vi "server.vi"() -> ()   [LabVIEW 2013, in "Experiment.lvclass"]
uses:
  Experiment.lvclass
  HSDIO/HSDIO_settings.ctl
  <instrlib>/niHSDIO/niHSDIO.llb/niHSDIO_ctl Trigger Script - trigID Values (Ring).ctl
  <instrlib>/niHSDIO/niHSDIO.llb/niHSDIO_ctl Trigger Source Values (Ring).ctl
  <instrlib>/niHSDIO/niHSDIO.llb/niHSDIO_ctl Trigger DigEdge - Edge Values (Ring).ctl
  <instrlib>/niHSDIO/niHSDIO.llb/niHSDIO_ctl Trigger DigLvl - Level Values (Ring).ctl
  HSDIO/waveform.ctl
  Camera/Hamamatsu_C9100-13/camera_setup.ctl
  <vilib>/Platform/TimedLoop/XDataNode/timing_clust.ctl
  <vilib>/Platform/TimedLoop/XDataNode/nitl_modes.ctl
  <vilib>/Platform/TimedLoop/XDataNode/wakeup.ctl
  Experiment.lvclass/Experiment.ctl
  HSDIO/HSDIO.lvclass
  Camera/Hamamatsu_C9100-13/Hamamatsu_C9100-13.lvclass
  Globals.vi
  <vilib>/platform/TimedLoop/XDataNode/XDataNode.xnode
  TCP_IP/TCP_IP.lvclass
  <vilib>/Platform/TimedLoop/XDataNode/XDNodeRunTimeDep.lvlib
panel:
  out "Log History":string
  in  "Tab Control":enum32{"HSDIO", "Camera"}(tab)=enum."Camera"
  out "HSDIO Settings":T1={"Enable HSDIO Pulses"=FALSE, "Resource Name"="PXI1Slot6", "Clock Rate"=20000000.0, "Array of Script Triggers"=[], "Pulse Generation Script"="script script1\n     Generate RedTrap_compress_temp\nend script", "Start Trigger"={"Wait for start trigger?"=FALSE, "source (PFI 0)"="PFI0", "edge (rising)"=12}, "Hardware alignment quantum\n(in samples)"=1, "Inital State"="", "Idle State"="", "Active Channels"="", "Array of Waveforms"=[]} {"Hardware alignment quantum\n(in samples)" min=1 step=1; "Array of Script Triggers"."level" items=["High Level"=34, "Low Level"=35]; "Array of Script Triggers"."edge" items=["Rising Edge"=12, "Falling Edge"=13]; "Start Trigger"."edge (rising)" items=["Rising Edge"=12, "Falling Edge"=13]; "Clock Rate" min=0.0 max=200000000.0 format="%.2p"}
  out "Camera Setup":T7={"Analog Gain (0-5)"=0, "Exposure Time"=0.01, "EM Gain (0-255)"=0, "Trigger Polarity"="ATP P", "External Trigger Mode"="EMD E", "Scan Speed"="SSP H", "External Trigger Source"="ESC B", "Scan Mode"="SMD N", "Super Pixel Binning\n(if enabled in Scan Mode)"="SPX 1", "Camera Sub-array acquisition region\n(if enabled in scan mode)"={"Left"=0, "Top"=0, "Width"=0, "Height"=0}, "Use camera?"=FALSE, "# image buffers"=100, "shots per measurement"=2, "Force images to U16"=FALSE, "Low Light Sensitivity"="LLS 0", "cooling"="CSW F", "fan"="FAN F", "Frame Grabber acquisition region"={"Left"=0, "Top"=0, "Right"=0, "Bottom"=0}} {"Frame Grabber acquisition region"."Bottom" max=512 step=1; "Frame Grabber acquisition region"."Right" max=512 step=1; "Frame Grabber acquisition region"."Top" max=512 step=1; "Frame Grabber acquisition region"."Left" max=512 step=1; "shots per measurement" min=0 step=1; "# image buffers" min=0 step=1; "Camera Sub-array acquisition region\n(if enabled in scan mode)"."Height" min=16 max=512 step=16; "Camera Sub-array acquisition region\n(if enabled in scan mode)"."Width" min=16 max=512 step=16; "Camera Sub-array acquisition region\n(if enabled in scan mode)"."Top" max=496 step=16; "Camera Sub-array acquisition region\n(if enabled in scan mode)"."Left" max=496 step=16; "Analog Gain (0-5)" max=5 step=1}
  in  "Clear Log":bool
  in  "Return fake test data":bool=TRUE
  out "Done":bool
  in  "Restart":bool
  out "Log":string
  in  "Stop":bool
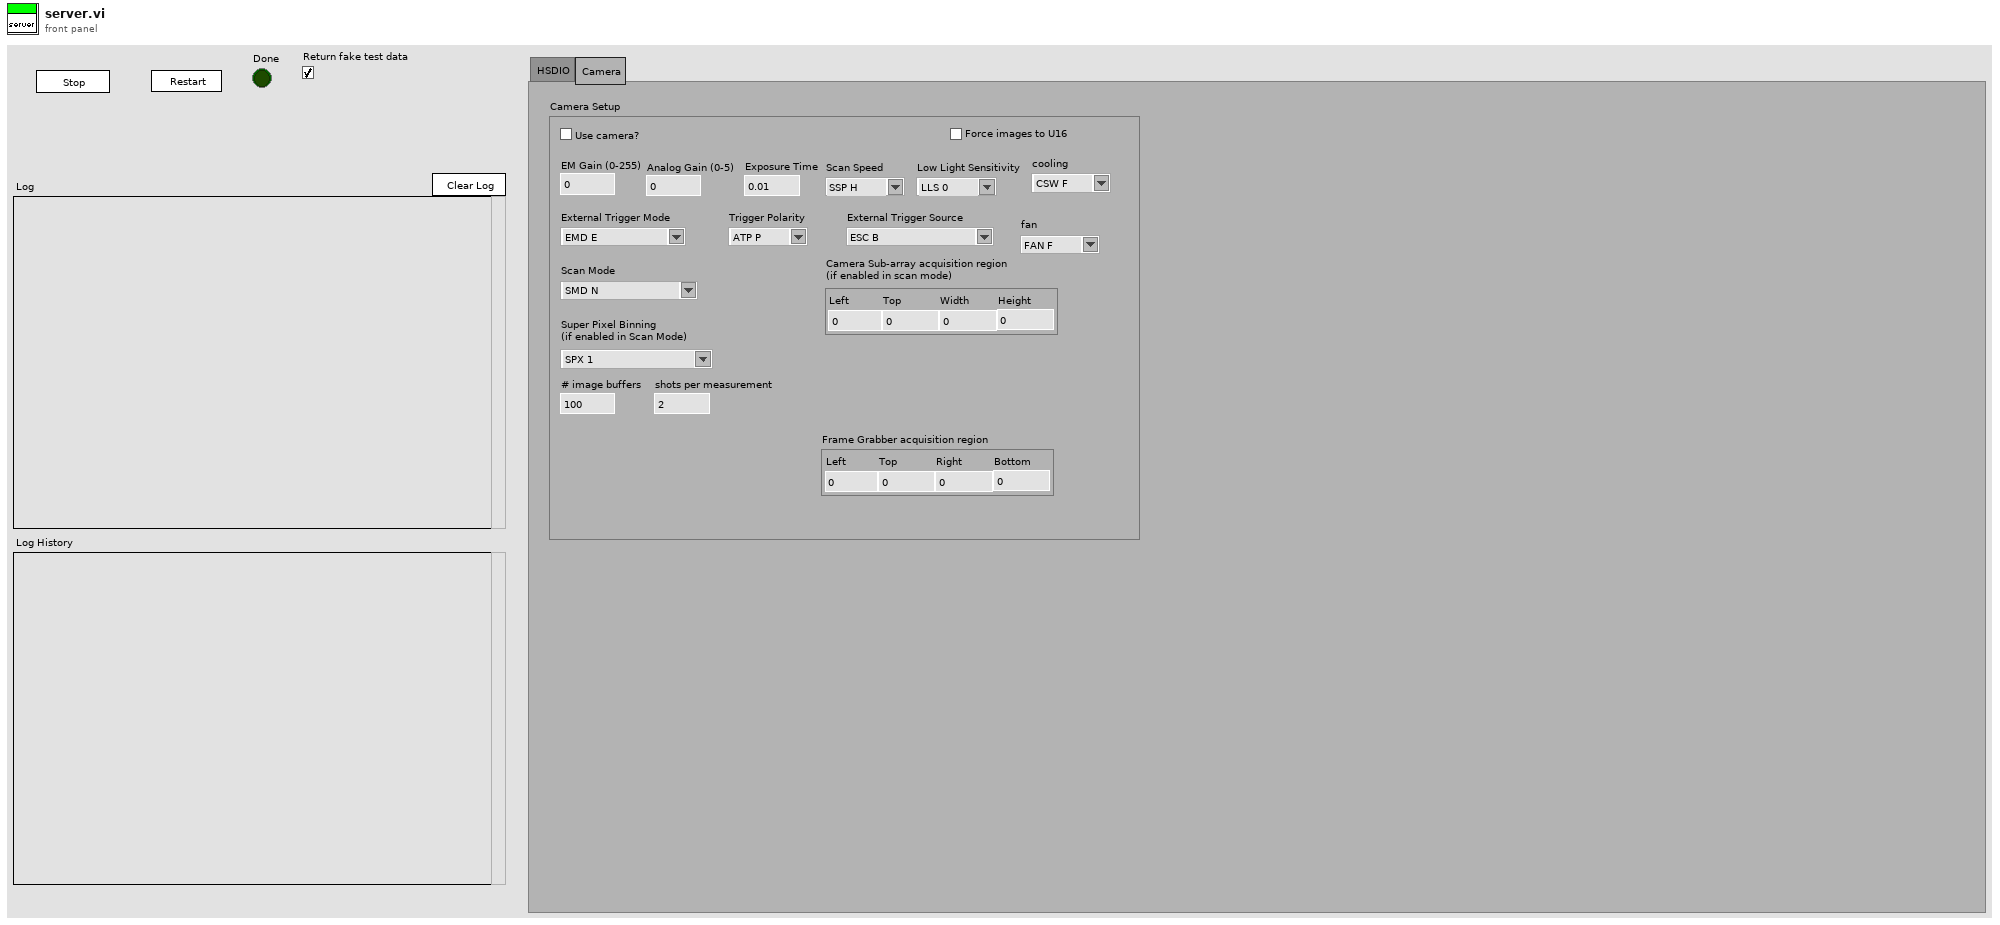
[diagram p1: front panel]
types:
  T1 = typedef "HSDIO.lvclass/HSDIO_settings.ctl" = cluster{"Enable HSDIO Pulses":bool, "Resource Name":refnum<k15>, "Clock Rate":dbl, "Array of Script Triggers":cluster{"trigger id (script trigger 0)":T2, "source (PFI 0)":T3, "Trigger Type":enum32{"Edge", "Level"}, "edge":T4, "level":T5}[], "Pulse Generation Script":string, "Start Trigger":cluster{"Wait for start trigger?":bool, "source (PFI 0)":T3, "edge (rising)":T4}, "Hardware alignment quantum\n(in samples)":u16, "Inital State":string, "Idle State":string, "Active Channels":string, "Array of Waveforms":T6[]}
  T2 = typedef "niHSDIO_ctl Trigger Script - trigID Values (Ring).ctl" = string
  T3 = typedef "niHSDIO_ctl Trigger Source Values (Ring).ctl" = string
  T4 = typedef "niHSDIO_ctl Trigger DigEdge - Edge Values (Ring).ctl" = i32
  T5 = typedef "niHSDIO_ctl Trigger DigLvl - Level Values (Ring).ctl" = i32
  T6 = typedef "HSDIO.lvclass/waveform.ctl" = cluster{"name":string, "transitions":u32[], "states":u8[][]}
  T7 = typedef "Hamamatsu_C9100-13.lvclass/camera_setup.ctl" = cluster{"Analog Gain (0-5)":u8, "Exposure Time":dbl, "EM Gain (0-255)":u8, "Trigger Polarity":string, "External Trigger Mode":string, "Scan Speed":string, "External Trigger Source":string, "Scan Mode":string, "Super Pixel Binning\n(if enabled in Scan Mode)":string, "Camera Sub-array acquisition region\n(if enabled in scan mode)":cluster{"Left":u16, "Top":u16, "Width":u16, "Height":u16}, "Use camera?":bool, "# image buffers":i32, "shots per measurement":i32, "Force images to U16":bool, "Low Light Sensitivity":string, "cooling":string, "fan":string, "Frame Grabber acquisition region":cluster{"Left":i32, "Top":i32, "Right":i32, "Bottom":i32}}
  T8 = typedef "XDNodeRunTimeDep.lvlib/timing_clust.ctl" = cluster{"Expected End [f-1]":u64, "Actual End [f-1]":u64, "Finished Late? [f-1]":bool, "Expected End [i-1]":u64, "Actual End [i-1]":u64, "Finished Late? [i-1]":bool, "Expected Start [i]":u64, "Actual Start [i]":u64, "Expected Start [f]":u64, "Actual Start [f]":u64, "Source Name":string, "Structure Name":string, "Period":i64, "Deadline":i64, "Offset":i64, "Start":i64, "Priority":i32, "Timeout":i32, "Mode":T9, "Wakeup Reason":T10, "Error":errorcluster, "Source Type":string, "Secondary Source Type":string, "Global End Time":u64, "Global Start Time":u64, "Frame Duration":u64, "Iteration Duration":u64, "Assigned CPU":i32, "I/O Scan Engine Mode":u32}
  T9 = typedef "XDNodeRunTimeDep.lvlib/nitl_modes.ctl" = enum32{"No Change", "Process missed periods, maintain original phase", "Discard missed periods, maintain original phase", "Process missed periods, ignore original phase", "Discard missed periods, ignore original phase"}
  T10 = typedef "XDNodeRunTimeDep.lvlib/wakeup.ctl" = enum32{"Normal", "Aborted", "Asynchronous wakeup", "Timing source error", "Timed loop error", "Timeout"}
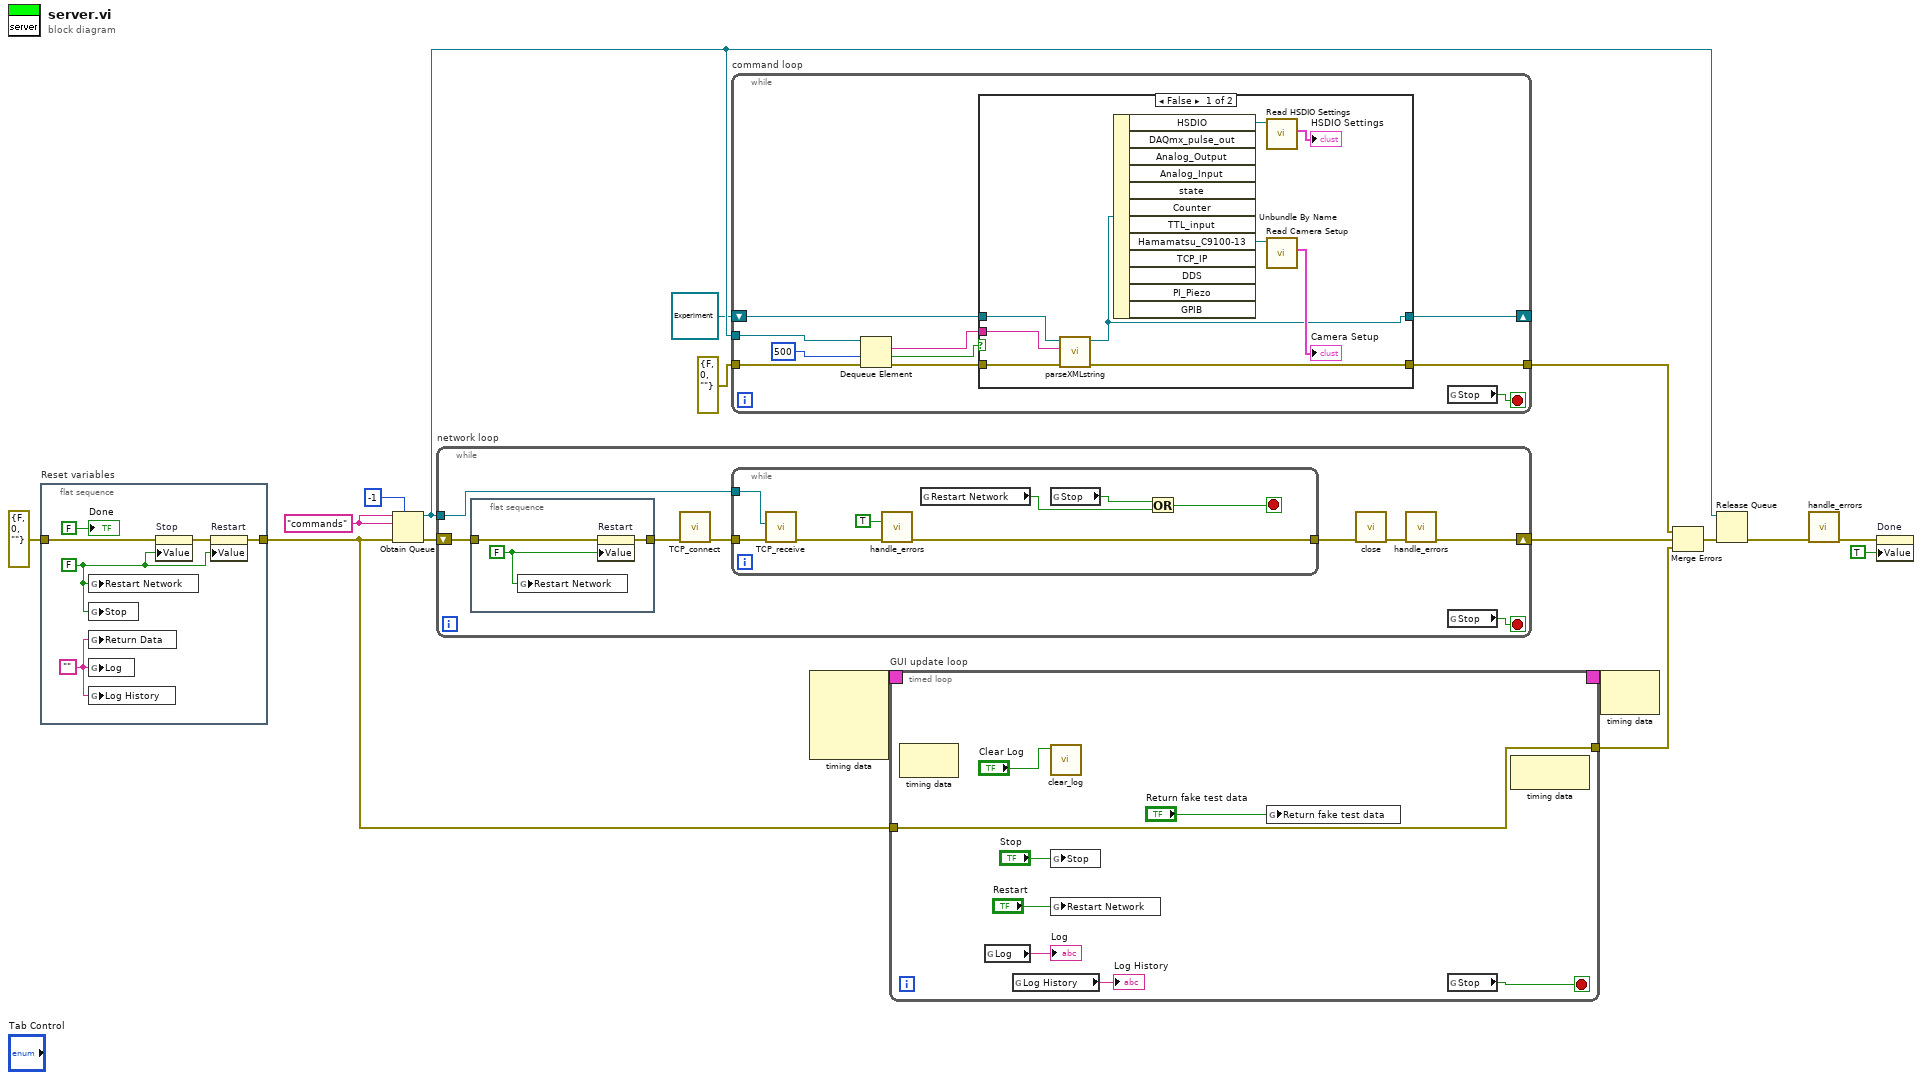
[diagram p0: block diagram]
diagram:
  w17 = "commands" ("name (unnamed)")
  n1 = flat-sequence "Reset variables" {
    tunnel: [w19] -> w6
    tunnel: errorcluster {"status"=FALSE, "code"=0, "source"=""} ("error in (no error)") -> [w21]
    frame #0 {
      w18 = ""
      w20 = FALSE ("Stop")
      n2 = global write "Globals.vi" "Restart Network"(w20) -> ()
      n3 = global write "Globals.vi" "Stop"(w20) -> ()
      n4 = global write "Globals.vi" "Return Data"(w18) -> ()
      n5 = global write "Globals.vi" "Log"(w18) -> ()
      n6 = global write "Globals.vi" "Log History"(w18) -> ()
      n7 = property on="Stop" class="Bool (strict)"(error in=w21, "Value"=w20) -> (error out=w23:errorcluster)  [unwired: 1 in, 1 out]
      n8 = property on="Restart" class="Bool (strict)"(error in=w23, "Value"=w20) -> (error out=w19:errorcluster)  [unwired: 1 in, 1 out]
      "Done" <- FALSE ("Done")
    }
  }
  n9 = Obtain Queue(max queue size (-1, unlimited)=-1, name (unnamed)=w17, element data type=w17, error in (no error)=w6) -> (queue out=w10:refnum<queue>, error out=w16:errorcluster)  [unwired: 1 in, 1 out]
  n10 = while "network loop" {
    shift-right: [w31] -> w9
    shift-left: w16 -> [w24]
    tunnel: w10 -> [w30]
    stop <- w28 stop-if-true
    n11 = flat-sequence {
      tunnel: [w33] -> w25
      tunnel: w24 -> [w34]
      frame #0 {
        w32 = FALSE ("Restart")
        n12 = global write "Globals.vi" "Restart Network"(w32) -> ()
        n13 = property on="Restart" class="Bool (strict)"(error in=w34, "Value"=w32) -> (error out=w33:errorcluster)  [unwired: 1 in, 1 out]
      }
    }
    n14 = call "TCP_connect.vi"("error in (no error)"=w25) -> ("error out"=w26:errorcluster)  [unwired: 10 in]
    n15 = while {
      tunnel: w26 -> [w40]
      tunnel: [w42] -> w29
      tunnel: w30 -> [w41]
      stop <- w39 stop-if-true
      n16 = call "TCP_receive.vi"("error in (no error)"=w40, "queue"=w41) -> ("error out"=w36:errorcluster)  [unwired: 9 in]
      n17 = call "handle_errors.vi"("Restart Network"=TRUE, "error in (no error)"=w36) -> ("error out"=w42:errorcluster)  [unwired: 13 in]
      n18 = global read "Globals.vi" "Restart Network"() -> (w37:bool)
      n19 = global read "Globals.vi" "Stop"() -> (w38:bool)
      n20 = Or(x=w38, y=w37) -> (x .or. y?=w39:bool)
    }
    n21 = call "close.vi"("error in (no error)"=w29) -> ("error out"=w27:errorcluster)  [unwired: 10 in]
    n22 = call "handle_errors.vi"("error in (no error)"=w27) -> ("error out"=w31:errorcluster)  [unwired: 14 in]
    n23 = global read "Globals.vi" "Stop"() -> (w28:bool)
  }
  n24 = while "command loop" {
    tunnel: w10 -> [w52]
    tunnel: errorcluster {"status"=FALSE, "code"=0, "source"=""} ("error constant") -> [w51]
    tunnel: [w43] -> w13
    shift-right: [w45] -> _
    shift-left: refnum<class "Experiment.lvclass"> refnum ("Experiment.lvclass") -> [w46]
    stop <- w44 stop-if-true
    n25 = Dequeue Element(queue=w52, timeout in ms (-1)=500, error in (no error)=w51) -> (element=w48:string, timed out?=w49:bool, error out=w50:errorcluster)  [unwired: 1 out]
    n26 = case shown="False" w49 {
      tunnel: [w61 w63] -> w43
      tunnel: w50 -> [w58 w63]
      tunnel: w48 -> [w60 _]
      tunnel: w46 -> [w59 w62]
      tunnel: [w53 w62] -> w45
      frame False {
        n27 = call "parseXMLstring.vi"("error in (no error)"=w58, "Node Value"=w60, "Experiment.lvclass (in)"=w59) -> ("error out"=w61:errorcluster, "Experiment.lvclass"=w53:refnum<class "Experiment.lvclass">)  [unwired: 7 in]
        n28 = Unbundle By Name(w53) -> ("HSDIO"=w57:refnum<class "HSDIO.lvclass">, "Hamamatsu_C9100-13"=w55:refnum<class "Hamamatsu_C9100-13.lvclass">)  [unwired: 10 out]
        n29 = call-dynamic "Read HSDIO Settings.vi"("HSDIO in"=w57) -> ("HSDIO Settings"=→"HSDIO Settings":T1)  [unwired: 5 in, 5 out]
        n30 = call-dynamic "Read Camera Setup.vi"("Hamamatsu_C9100-13 in"=w55) -> ("Camera Setup"=→"Camera Setup":T7)  [unwired: 8 in, 2 out]
      }
      frame True {
      }
    }
    n31 = global read "Globals.vi" "Stop"() -> (w44:bool)
  }
  n32 = node-c288() -> (w2:T8)  [unwired: 4 in]
  n33 = timed-loop "GUI update loop" {
    tunnel: w6 -> [w67]
    tunnel: [w67] -> w5
    timing: w2 -> [_]
    timing-out: [_] -> w1
    stop <- w68 stop-if-true
    n34 = node-c288() -> ()  [unwired: 1 in, 1 out]
    n35 = global read "Globals.vi" "Log"() -> (→"Log":string)
    n36 = global read "Globals.vi" "Log History"() -> (→"Log History":string)
    n37 = call "clear_log.vi"("clear log?"="Clear Log") -> ()  [unwired: 10 in, 1 out]
    n38 = global write "Globals.vi" "Stop"("Stop") -> ()
    n39 = global write "Globals.vi" "Restart Network"("Restart") -> ()
    n40 = global write "Globals.vi" "Return fake test data"("Return fake test data") -> ()
    n41 = global read "Globals.vi" "Stop"() -> (w68:bool)
    n42 = node-c288() -> ()  [unwired: 1 in, 1 out]
  }
  n43 = node-c288(w1) -> ()  [unwired: 1 out]
  n44 = Merge Errors(w13, w9, w5) -> (w12:errorcluster)
  n45 = Release Queue(queue=w10, error in (no error)=w12) -> (error out=w11:errorcluster)  [unwired: 1 in, 2 out]
  n46 = call "handle_errors.vi"("error in (no error)"=w11) -> ("error out"=w4:errorcluster)  [unwired: 14 in]
  n47 = property on="Done" class="Bool (strict)"(error in=w4, "Value"=TRUE ("Done")) -> ()  [unwired: 1 in, 2 out]
